vi "Panel.vi"(11 "Square Field Panel in":refnum<class "Square Field Panel.lvclass">) -> ()   [LabVIEW 2020, in "SB App.lvlib" / "Square Field Panel.lvclass"]
uses:
  Square Field Panel.lvclass
  C:/Program Files (x86)/National Instruments/LabVIEW 2020/vi.lib/IlluminatedG/IG OOPanel/OOPanel/Panel/Panel.lvclass
  <vilib>/IlluminatedG/IG OOPanel/OOPanel/Panel/Basic UI State.ctl
  <vilib>/IlluminatedG/IG OOPanel/OOPanel/Panel/Panel.lvclass
  <vilib>/IlluminatedG/IG OOPanel/OOPanel/OOPanel.lvlib
panel:
  out "Team Field":i32[][](graph)
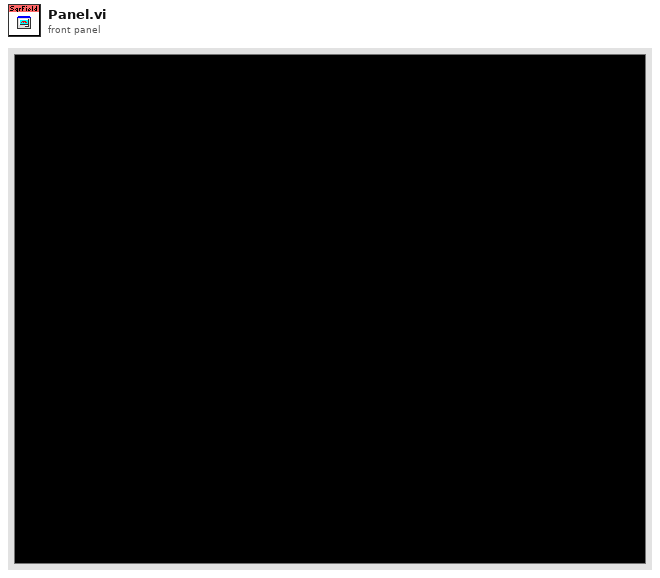
[diagram p1: front panel]
types:
  T1 = typedef "OOPanel.lvlib/Panel.lvclass/Basic UI State.ctl" = enum16{"Init", "Run", "Close"}
  T2 = typedef "OOPanel.lvlib/Panel.lvclass/Panel Events.ctl" = cluster{"Visbility":refnum<user-event>, "Close":refnum<user-event>}
  T3 = typedef "OOPanel.lvlib/Panel.lvclass/Visibility State.ctl" = enum16{"Idle", "Closed", "Hidden", "Visible", "Subpanel"}
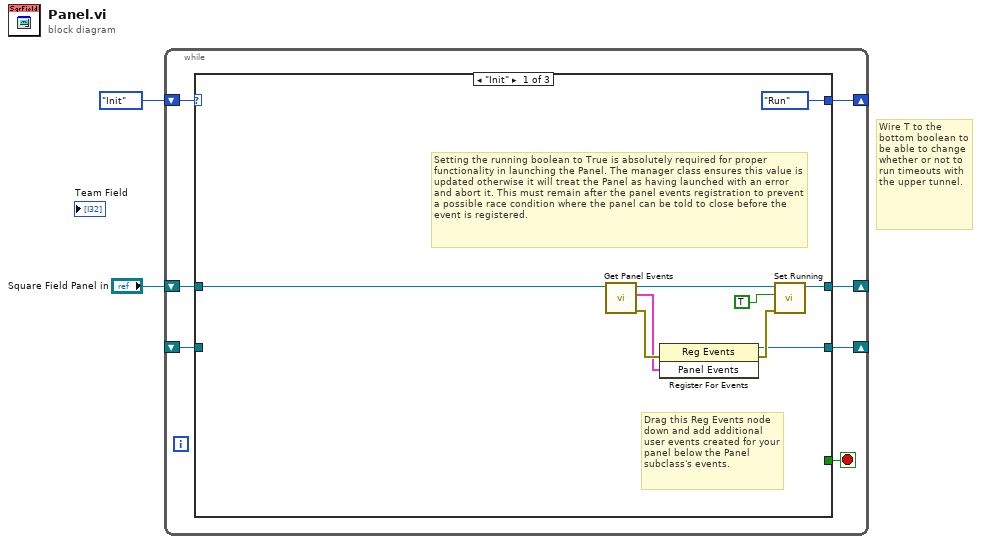
[diagram p0: block diagram]
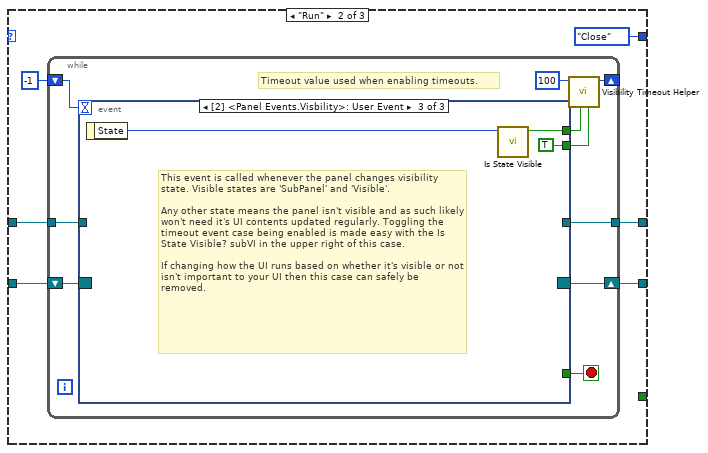
[diagram p2: hidden frame]
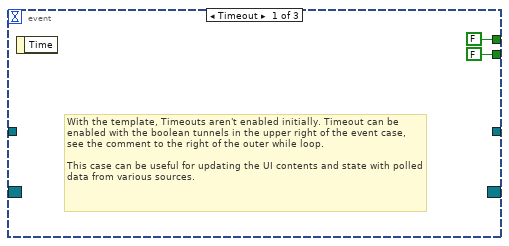
[diagram p3: hidden frame]
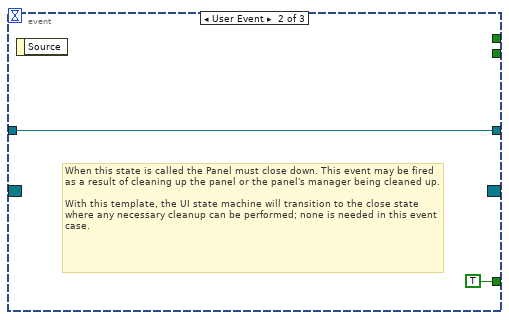
[diagram p4: hidden frame]
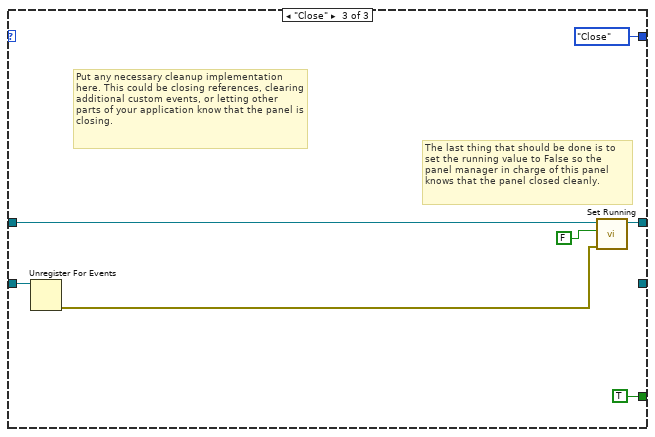
[diagram p5: hidden frame]
diagram:
  # "Wire T to the bottom boolean to be able to change whether or not to run timeouts with the upper tunnel."
  n1 = while {
    shift-right: [w8] -> _
    shift-left: _ -> [w9]
    shift-right: [w6] -> _
    shift-left: Basic_UI_State."Init" ("Basic UI State") -> [w7]
    shift-right: [w4] -> _
    shift-left: "Square Field Panel in" -> [w3]
    stop <- w5 stop-if-true
    n2 = case shown="\"Init\"" w7 {
      tunnel: w9 -> [_ w24 w44]
      tunnel: [w12 w22 _] -> w8
      tunnel: [Basic_UI_State."Run" ("Basic UI State") Basic_UI_State."Close" ("Basic UI State") Basic_UI_State."Close" ("Basic UI State")] -> w6
      tunnel: [_ _ TRUE] -> w5
      tunnel: [w11 w19 w42] -> w4
      tunnel: w3 -> [w10 w20 w43]
      frame "Init" {
        # "Setting the running boolean to True is absolutely required for proper functionality in launching the Panel. The manager class ensures this value is updated otherwise it will treat the Panel as having launched with an error and abort it. This must remain after the panel events registration to prevent a possible race condition where the panel can be told to close before the event is registered."
        # "Drag this Reg Events node down and add additional user events created for your panel below the Panel subclass's events."
        n3 = call <vilib>:"Get Panel Events.vi"("Panel in"=w10) -> ("error out"=w18:errorcluster, "Panel Events"=w14:T2, "Panel out"=w15:refnum<class "Square Field Panel.lvclass">)  [unwired: 8 in]
        n4 = register-events(error in=w18, w14) -> (reference out=w12:refnum<event-registration>, error out=w16:errorcluster)  [unwired: 1 in]
        n5 = call <vilib>:"Set Running.vi"("error in (no error)"=w16, "Running"=TRUE, "Panel in"=w15) -> ("Panel out"=w11:refnum<class "Square Field Panel.lvclass">)  [unwired: 7 in, 1 out]
      }
      frame "Run" {
        n6 = while {
          shift-right: [w30] -> w22
          shift-left: w24 -> [w31]
          shift-right: [w33] -> _
          shift-left: -1 ("Timeout") -> [w32]
          tunnel: w20 -> [w26]
          tunnel: [w25] -> w19
          stop <- w27 stop-if-true
          # "Timeout value used when enabling timeouts."
          n7 = event shown="[2] <Panel Events.Visbility>: User Event" {
            selector: w31 -> [_ _ _]
            dyn-events: [_ _ _] -> w30
            timeout: w32 -> [_ _ _]
            tunnel: [FALSE _ w40] -> w29
            tunnel: [FALSE _ TRUE] -> w28
            tunnel: [_ TRUE _] -> w27
            tunnel: w26 -> [_ w37 _]
            tunnel: [_ w37 _] -> w25
            event Timeout {
              # "With the template, Timeouts aren't enabled initially. Timeout can be enabled with the boolean tunnels in the upper right of the event case, see the comment to the right of the outer while loop.\n\nThis case can be useful for updating the UI contents and state with polled data from various sources."
              n8 = event-data() -> ()  [unwired: 1 in, 1 out]
            }
            event User Event {
              # "When this state is called the Panel must close down. This event may be fired as a result of cleaning up the panel or the panel's manager being cleaned up.\n\nWith this template, the UI state machine will transition to the close state where any necessary cleanup can be performed; none is needed in this event case."
              n9 = event-data() -> ()  [unwired: 1 in, 1 out]
            }
            event User Event {
              # "This event is called whenever the panel changes visibility state. Visible states are 'SubPanel' and 'Visible'.\n\nAny other state means the panel isn't visible and as such likely won't need it's UI contents updated regularly. Toggling the timeout event case being enabled is made easy with the Is State Visible? subVI in the upper right of this case.\n\nIf changing how the UI runs based on whether it's visible or not isn't important to your UI then this case can safely be removed."
              n10 = event-data() -> ("State"=w41:T3)  [unwired: 1 in]
              n11 = call <vilib>:"Is State Visible.vi"("Visibility"=w41) -> ("Visible"=w40:bool)  [unwired: 10 in]
            }
          }
          n12 = call <vilib>:"Visibility Timeout Helper.vi"("Update?"=w28, "Use Timeout?"=w29, "Visible Timeout mS"=100) -> ("Timeout"=w33:i32)  [unwired: 8 in]
        }
      }
      frame "Close" {
        # "Put any necessary cleanup implementation here. This could be closing references, clearing additional custom events, or letting other parts of your application know that the panel is closing."
        # "The last thing that should be done is to set the running value to False so the panel manager in charge of this panel knows that the panel closed cleanly."
        n13 = Unregister For Events(event registration refnum=w44) -> (error out=w46:errorcluster)  [unwired: 1 in]
        n14 = call <vilib>:"Set Running.vi"("error in (no error)"=w46, "Running"=FALSE, "Panel in"=w43) -> ("Panel out"=w42:refnum<class "Square Field Panel.lvclass">)  [unwired: 7 in, 1 out]
      }
    }
  }
